vi "P8.vi"() -> ()   [LabVIEW 2019]
panel:
  out "C":bool
  out "B":bool
  out "A":bool
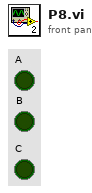
[diagram p1: front panel]
types:
  T1 = typedef "Semaphore RefNum" = refnum<k1>
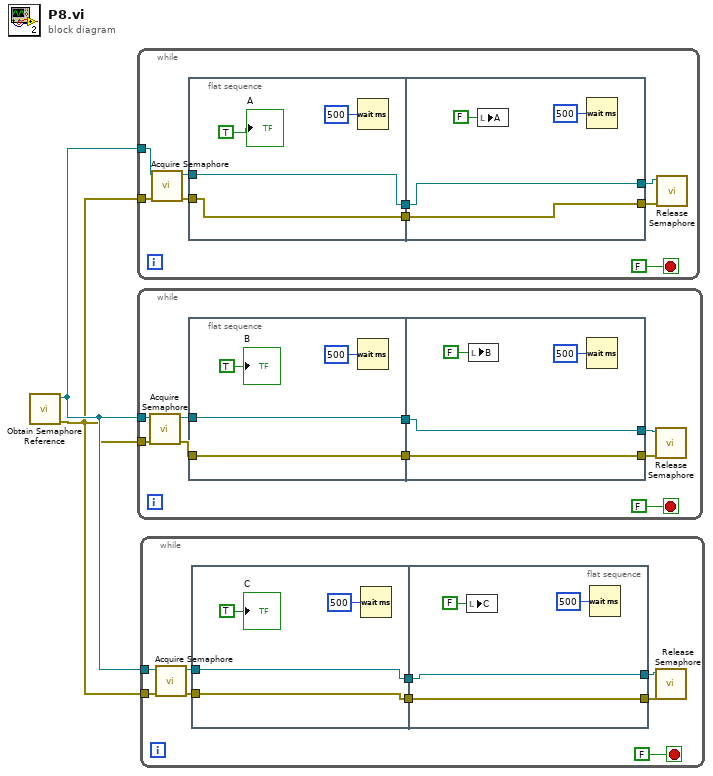
[diagram p0: block diagram]
diagram:
  n1 = call <vilib>:"Obtain Semaphore Reference.vi"() -> ("error out"=w1:errorcluster, "semaphore"=w2:T1)  [unwired: 5 in, 1 out]
  n2 = while {
    tunnel: w2 -> [w10]
    tunnel: w1 -> [w6]
    stop <- FALSE stop-if-true
    n3 = call <vilib>:"Acquire Semaphore.vi"("error in (no error)"=w6, "semaphore"=w10) -> ("error out"=w5:errorcluster, "semaphore out"=w8:T1)  [unwired: 3 in, 1 out]
    n4 = flat-sequence {
      tunnel: [w13] -> w9
      tunnel: w8 -> [w13]
      tunnel: w5 -> [w12]
      tunnel: [w12] -> w4
      tunnel: w9 -> [w17]
      tunnel: [w17] -> w7
      tunnel: w4 -> [w16]
      tunnel: [w16] -> w3
      frame #0 {
        n5 = Wait (ms)(milliseconds to wait=u32 500) -> ()  [unwired: 1 out]
        "A" <- TRUE ("A")
      }
      frame #1 {
        n6 = local write "A"(FALSE ("A")) -> ()
        n7 = Wait (ms)(milliseconds to wait=u32 500) -> ()  [unwired: 1 out]
      }
    }
    n8 = call <vilib>:"Release Semaphore.vi"("error in (no error)"=w3, "semaphore"=w7) -> ()  [unwired: 4 in, 2 out]
  }
  n9 = while {
    tunnel: w2 -> [w27]
    tunnel: w1 -> [w23]
    stop <- FALSE stop-if-true
    n10 = call <vilib>:"Acquire Semaphore.vi"("error in (no error)"=w23, "semaphore"=w27) -> ("error out"=w21:errorcluster, "semaphore out"=w26:T1)  [unwired: 3 in, 1 out]
    n11 = flat-sequence {
      tunnel: w26 -> [w30]
      tunnel: [w30] -> w25
      tunnel: [w29] -> w22
      tunnel: w21 -> [w29]
      tunnel: w25 -> [w34]
      tunnel: [w34] -> w24
      tunnel: w22 -> [w33]
      tunnel: [w33] -> w20
      frame #0 {
        n12 = Wait (ms)(milliseconds to wait=u32 500) -> ()  [unwired: 1 out]
        "B" <- TRUE ("A")
      }
      frame #1 {
        n13 = local write "B"(FALSE ("A")) -> ()
        n14 = Wait (ms)(milliseconds to wait=u32 500) -> ()  [unwired: 1 out]
      }
    }
    n15 = call <vilib>:"Release Semaphore.vi"("error in (no error)"=w20, "semaphore"=w24) -> ()  [unwired: 4 in, 2 out]
  }
  n16 = while {
    tunnel: w2 -> [w44]
    tunnel: w1 -> [w40]
    stop <- FALSE stop-if-true
    n17 = call <vilib>:"Acquire Semaphore.vi"("error in (no error)"=w40, "semaphore"=w44) -> ("error out"=w38:errorcluster, "semaphore out"=w42:T1)  [unwired: 3 in, 1 out]
    n18 = flat-sequence {
      tunnel: [w47] -> w43
      tunnel: w42 -> [w47]
      tunnel: [w46] -> w39
      tunnel: w38 -> [w46]
      tunnel: w43 -> [w51]
      tunnel: [w51] -> w41
      tunnel: w39 -> [w50]
      tunnel: [w50] -> w37
      frame #0 {
        n19 = Wait (ms)(milliseconds to wait=u32 500) -> ()  [unwired: 1 out]
        "C" <- TRUE ("A")
      }
      frame #1 {
        n20 = local write "C"(FALSE ("A")) -> ()
        n21 = Wait (ms)(milliseconds to wait=u32 500) -> ()  [unwired: 1 out]
      }
    }
    n22 = call <vilib>:"Release Semaphore.vi"("error in (no error)"=w37, "semaphore"=w41) -> ()  [unwired: 4 in, 2 out]
  }
